vi "Save Configuration to file.vi"() -> ()   [LabVIEW 2012]
panel:
  out "cancelled":bool
  out "refnum out":refnum<file>
  in  "VISA resource name":refnum<visa-resource-name>="COM1"
  in  "Addr (0-15)":i8=1 min=0 max=15 step=1
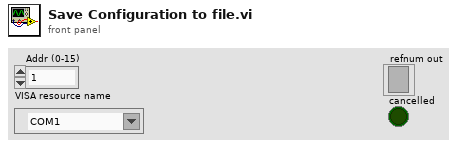
[diagram p1: front panel]
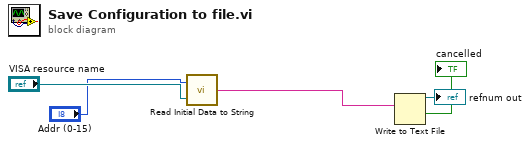
[diagram p0: block diagram]
diagram:
  n1 = call "Read Initial Data to String.vi"("VISA resource name"="VISA resource name", "Addr (0-15)"="Addr (0-15)") -> ("Data"=w3:string)
  n2 = Write to Text File(text=w3) -> (refnum out=→"refnum out":refnum<file>, cancelled=→"cancelled":bool)  [unwired: 3 in, 1 out]
